vi "rsscope Configure Display Update.vi"(8 "error in (no error)":errorcluster, 10 "Display In Remote (Off)":bool, 11 "VISA resource name":refnum<visa-resource-name>) -> (0 "error out":errorcluster, 3 "VISA resource name out":refnum<visa-resource-name>)   [LabVIEW 2018]
doc: "This VI switches on or off the update of all display elements during remote control.\n\nNote:\n- The best performance is obtained when the display output is switched off during remote control.\n\nAttribute:\nRSSCOPE_ATTR_DISPLAY_UPDATE\n\nRemote-control command:\nSYSTem:DISPlay:UPDate"
uses:
  Instance           1 37Saved   rsscope Configure Persistence .vi
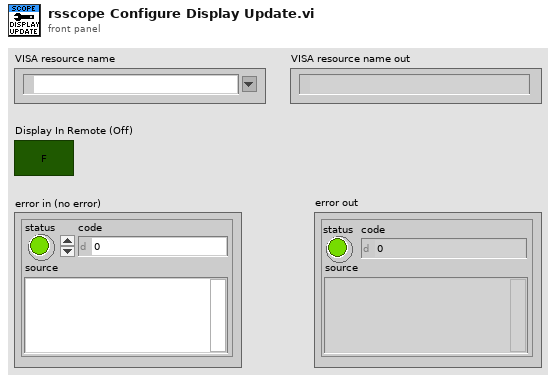
[diagram p1: front panel]
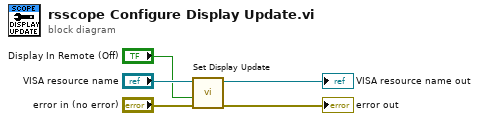
[diagram p0: block diagram]
diagram:
  n1 = call "Set Display Update"("error in (no error)"="error in (no error)", "Display Update (OFF)"="Display In Remote (Off)", "instrument handle"="VISA resource name") -> ("error out"=→"error out":errorcluster, "instrument handle out"=→"VISA resource name out":refnum<visa-resource-name>)  [unwired: 7 in]
